vi "Define Relation.vi"(10 "Relation Definition":T1, 11 "Relation in":refnum<class "Relation.lvclass">) -> (3 "Relation out":refnum<class "Relation.lvclass">)   [LabVIEW 2020, in "Conditum.lvlib" / "Columns.lvlib" / "Relation.lvclass"]
uses:
  Relation.lvclass
  C:/dev/lv20CE/lv-conditum/Conditum/Columns/Type/Type.lvclass
  Relation Definition.ctl
  Type/Definition.ctl
  Relation Info.ctl
  Relation Mapping.ctl
  Field Type.ctl
  Attributes.ctl
  Type/Type.lvclass/Type.ctl
  Relation.lvclass/Relation.ctl
  Type/Type.lvclass
  Conditum.lvlib
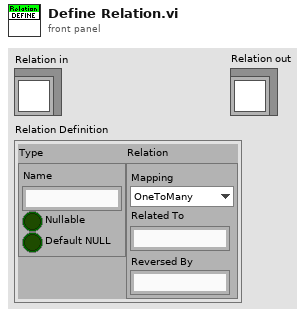
[diagram p1: front panel]
types:
  T1 = typedef "Conditum.lvlib/Columns.lvlib/Relation.lvclass/Relation Definition.ctl" = cluster{"Type":T2, "Relation":T3}
  T2 = typedef "Conditum.lvlib/Columns.lvlib/Type.lvclass/Definition.ctl" = cluster{"Name":string, "Nullable":bool, "Default NULL":bool}
  T3 = typedef "Conditum.lvlib/Relation Info.ctl" = cluster{"Mapping":T4, "Related To":string, "Reversed By":string}
  T4 = typedef "Conditum.lvlib/Relation Mapping.ctl" = enum16{"OneToMany", "ManyToOne", "ManyToMany", "OneToOne"}
  T5 = typedef "Conditum.lvlib/Field Type.ctl" = enum16{"None", "ID", "Boolean", "Integer", "Double", "Timestamp", "String", "Text", "Entity"}
  T6 = typedef "Conditum.lvlib/Attributes.ctl" = cluster{"Primary Key":bool, "Unique":bool, "Foreign Key":bool, "Auto Increment":bool}
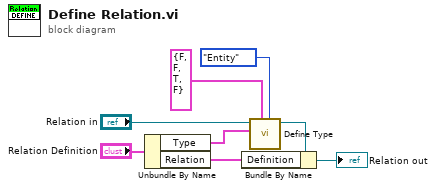
[diagram p0: block diagram]
diagram:
  n1 = Unbundle By Name("Relation Definition") -> ("Type"=w6:T2, "Relation"=w4:T3)
  n2 = call "Define Type.vi"("Type"=Field_Type."Entity", "Attributes"=T6 {"Primary Key"=FALSE, "Unique"=FALSE, "Foreign Key"=TRUE, "Auto Increment"=FALSE}, "Definition"=w6, "Type in"="Relation in") -> ("Type out"=w3:refnum<class "Relation.lvclass">)  [unwired: 7 in]
  n3 = Bundle By Name(cluster=w3, "Definition"=w4) -> (→"Relation out":refnum<class "Relation.lvclass">)
